vi "Multi Latch.vi"(8 "4":bool, 9 "3":bool, 10 "2":bool, 11 "1":bool) -> (0 "4":bool, 1 "3":bool, 2 "2":bool, 3 "1":bool)   [LabVIEW 2014]
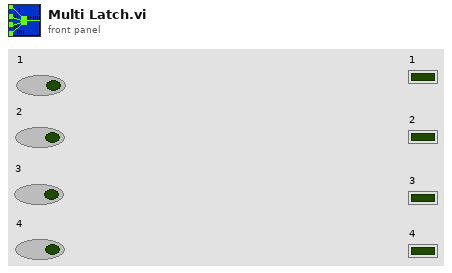
[diagram p1: front panel]
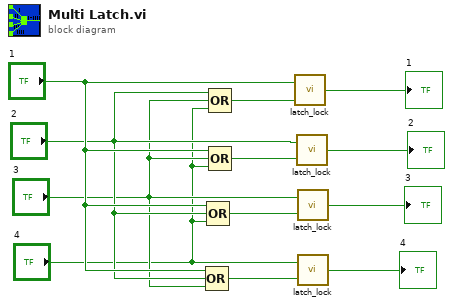
[diagram p0: block diagram]
diagram:
  n1 = Compound Arithmetic op=OR("1", "2", "3") -> (w10:bool)
  n2 = Compound Arithmetic op=OR("1", "2", "4") -> (w11:bool)
  n3 = Compound Arithmetic op=OR("2", "3", "4") -> (w1:bool)
  n4 = Compound Arithmetic op=OR("1", "3", "4") -> (w12:bool)
  n5 = call "latch_lock.vi"("Reset"=w1, "GO!"="1") -> ("ON"=→"1":bool)
  n6 = call "latch_lock.vi"("Reset"=w12, "GO!"="2") -> ("ON"=→"2":bool)
  n7 = call "latch_lock.vi"("Reset"=w11, "GO!"="3") -> ("ON"=→"3":bool)
  n8 = call "latch_lock.vi"("Reset"=w10, "GO!"="4") -> ("ON"=→"4":bool)
